vi "Read and conv. to number.vi"(8 "error in":errorcluster, 9 "Bytes at port <X or = 0?":bool, 10 "Num. of Bytes at Port":u32, 11 "port":refnum<visa-resource-name>) -> (0 "error out":errorcluster, 3 "Temper.":dbl, 4 "Bytes at port <X or = 0? 2":bool)   [LabVIEW 2013]
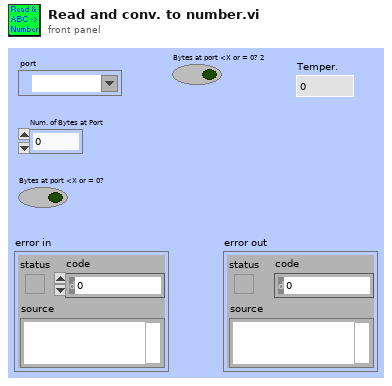
[diagram p1: front panel]
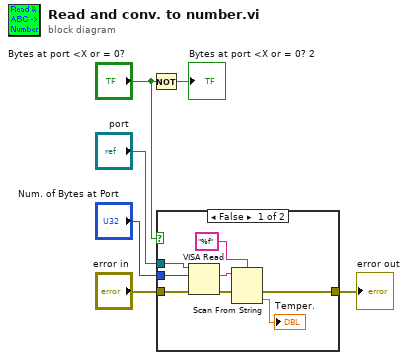
[diagram p0: block diagram]
diagram:
  n1 = Not(x="Bytes at port <X or = 0?") -> (.not. x?=→"Bytes at port <X or = 0? 2":bool)
  n2 = case shown="False" "Bytes at port <X or = 0?" {
    tunnel: [w10 w15] -> w5
    tunnel: "Num. of Bytes at Port" -> [w14 _]
    tunnel: "port" -> [w13 _]
    tunnel: "error in" -> [w12 w15]
    frame False {
      n3 = VISA Read(VISA resource name=w13, byte count=w14, error in (no error)=w12) -> (read buffer=w7:string, error out=w11:errorcluster)  [unwired: 2 out]
      n4 = Scan From String(format string="%f", input string=w7, error in=w11) -> (error out=w10:errorcluster, output 1=→"Temper.":dbl)  [unwired: 2 in, 2 out]
    }
    frame True {
    }
  }
  "error out" <- w5
